vi "Extract_HDF5_Files.vi"(10 "filenames":string[](array[string]), 11 "path":path) -> (2 "FileNames":string[](array[string]), 3 "Folders":path[](array[path]))   [LabVIEW 2018]
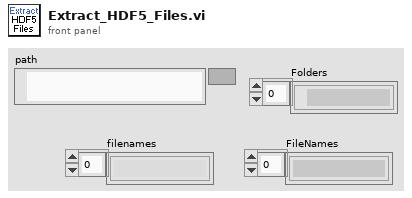
[diagram p1: front panel]
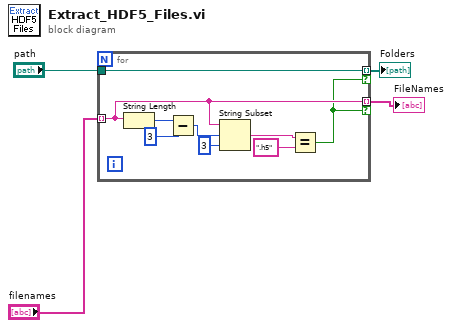
[diagram p0: block diagram]
diagram:
  n1 = for {
    tunnel: "filenames" -> [w7] mode=indexing
    tunnel: [w7] -> w4 mode=indexing if=w5
    tunnel: [w6] -> w1 mode=indexing if=w5
    tunnel: "path" -> [w6]
    n2 = String Length(string=w7) -> (length=w13:i32)
    n3 = Subtract(x=w13, y=3) -> (x-y=w11:i32)
    n4 = String Subset(string=w7, offset (0)=w11, length (rest)=3 ("length (rest)")) -> (substring=w9:string)
    n5 = Equal?(x=w9, y=".h5") -> (x = y?=w5:bool)
  }
  "FileNames" <- w4
  "Folders" <- w1
